vi "MOCKBEAR_Initialize.vi"(8 "error in (no error)":errorcluster, 11 "MOCKBEAR in":refnum<class "MOCKBEAR.lvclass">) -> (0 "error out":errorcluster, 3 "MOCKBEAR out":refnum<class "MOCKBEAR.lvclass">)   [LabVIEW 2021, in "MOCKBEAR.lvclass"]
uses:
  MOCKBEAR.lvclass
  MOCKBEAR.lvclass/MOCKBEAR.ctl
panel:
  out "output cluster":T1
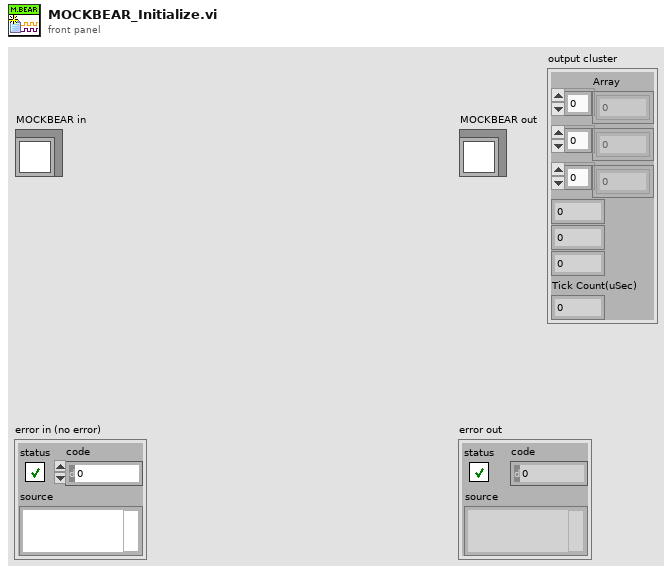
[diagram p1: front panel]
types:
  T1 = cluster{"Array":dbl[], dbl[], dbl[], dbl, dbl, i32, "Tick Count(uSec)":u32}
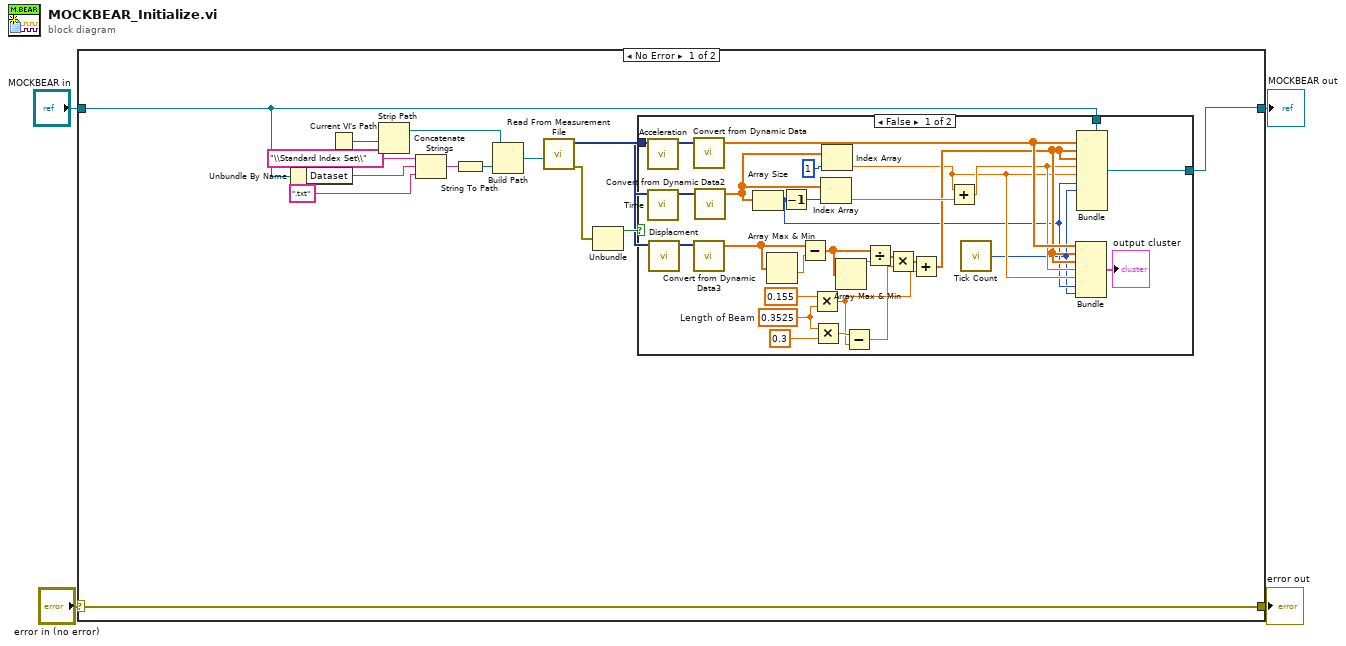
[diagram p0: block diagram]
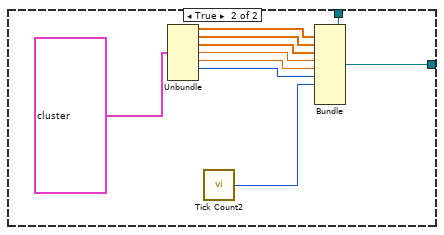
[diagram p2: hidden frame]
diagram:
  n1 = case shown="No Error" "error in (no error)" {
    selector: "error in (no error)" -> [w9 w59]
    tunnel: [w9 w59] -> w3
    tunnel: [w12 w58] -> w1
    tunnel: "MOCKBEAR in" -> [w13 w58]
    frame No Error {
      n2 = Unbundle By Name(w13) -> ("Dataset"=w16:string)
      n3 = Current VI's Path() -> (path=w6:path)
      n4 = Strip Path(path=w6) -> (stripped path=w5:path)  [unwired: 1 out]
      n5 = Concatenate Strings("\\Standard Index Set\\", w16, ".txt") -> (w11:string)
      n6 = String To Path(string=w11) -> (path=w14:path)
      n7 = Build Path(base path=w5, name or relative path=w14) -> (appended path=w18:path)
      n8 = call "Read From Measurement File"("Filename"=w18) -> ("error out"=w8:errorcluster, "Signals"=w17:dynamicdata)  [unwired: 5 in, 4 out]
      n9 = Unbundle(w8) -> ("status"=w7:bool)  [unwired: 2 out]
      n10 = case shown="False" w7 {
        tunnel: w17 -> [w47 _]
        tunnel: w13 -> [w46 w56]
        tunnel: [w45 w57] -> w12
        frame False {
          w36 = 0.3525  # Length of Beam
          n11 = call "Acceleration"("Signals"=w47) -> ("Signal Out"=w43:dynamicdata)  [unwired: 9 in, 1 out]
          n12 = call "Time"("Signals"=w47) -> ("Signal Out"=w42:dynamicdata)  [unwired: 9 in, 1 out]
          n13 = call "Displacment"("Signals"=w47) -> ("Signal Out"=w38:dynamicdata)  [unwired: 9 in, 1 out]
          n14 = call "Convert from Dynamic Data"("Dynamic Data Type"=w43) -> ("Array"=w25:dbl[])  [unwired: 3 in]
          n15 = call "Convert from Dynamic Data3"("Dynamic Data Type"=w38) -> ("Array"=w32:dbl[])  [unwired: 3 in]
          n16 = call "Convert from Dynamic Data2"("Dynamic Data Type"=w42) -> ("Array"=w40:dbl[])  [unwired: 3 in]
          n17 = Array Size(array=w40) -> (size(s)=w21:i32)
          n18 = Array Max & Min(array=w32) -> (min value=w34:dbl)  [unwired: 3 out]
          n19 = Decrement(x=w21) -> (x-1=w39:i32)
          n20 = Subtract(x=w32, y=w34) -> (x-y=w31:dbl[])
          n21 = Multiply(x=0.155, y=w36) -> (x*y=w27:dbl)
          n22 = Multiply(x=w36, y=0.3) -> (x*y=w28:dbl)
          n23 = Index Array(array=w40, index=w39) -> (element=w44:dbl)
          n24 = Index Array(array=w40, index=1) -> (element=w22:dbl)
          n25 = Array Max & Min(array=w31) -> (max value=w30:dbl)  [unwired: 3 out]
          n26 = Subtract(x=w28, y=w27) -> (x-y=w26:dbl)
          n27 = Divide(x=w31, y=w30) -> (x/y=w29:dbl[])
          n28 = Multiply(x=w29, y=w26) -> (x*y=w33:dbl[])
          n29 = Add(x=w33, y=w27) -> (x+y=w24:dbl[])
          n30 = Add(x=w22, y=w44) -> (x+y=w23:dbl)
          n31 = call "Tick Count"() -> ("Tick Count(uSec)"=w20:u32)
          n32 = Bundle("Array"=w25, w24, w24, w23, w22, w21, "Tick Count(uSec)"=w20) -> (→"output cluster":T1)  [unwired: 1 in]
          n33 = Bundle(cluster=w46, w25, w24, w24, w23, w22, w21, w20) -> (w45:refnum<class "MOCKBEAR.lvclass">)  [unwired: 3 in]
        }
        frame True {
          n34 = Unbundle(T1 {"Array"=array[210000 elements], array[210000 elements], array[210000 elements], 42.0, 0.0002, 210000, "Tick Count(uSec)"=1139227113} ("output cluster")) -> ("Array"=w53:dbl[], w52:dbl[], w51:dbl[], w50:dbl, w49:dbl, w48:i32)  [unwired: 1 out]
          n35 = call "Tick Count2"() -> ("Tick Count(uSec)"=w55:u32)
          n36 = Bundle(cluster=w56, w53, w52, w51, w50, w49, w48, w55) -> (w57:refnum<class "MOCKBEAR.lvclass">)  [unwired: 3 in]
        }
      }
    }
    frame Error {
    }
  }
  "error out" <- w3
  "MOCKBEAR out" <- w1
